vi "HFRR ADV v06.vi"() -> ()   [LabVIEW 2025] (continued)
1.510957261467722, 1.5101897326343034, 1.5103432384009872, 1.5098827211009362, 1.5114177787677732, 1.5108037557010383, 1.5104967441676709, 1.510957261467722, 1.5101897326343034, 1.5111107672344057, 1.5106502499343546, 1.5103432384009872, 1.5108037557010383, 1.5095757095675688, 1.5106502499343546, 1.5103432384009872, 1.5104967441676709, 1.5111107672344057, 1.5104967441676709, 1.5103432384009872, 1.5112642730010895, 1.5108037557010383, 1.5103432384009872, 1.5104967441676709, 1.5106502499343546, 1.5106502499343546, 1.5108037557010383, 1.5111107672344057, 1.5095757095675688, 1.5097292153342525, 1.5111107672344057, 1.5104967441676709, 1.5138738710347124, 1.5138738710347124, 1.5124923191345592, 1.5115712845344569, 1.510957261467722, 1.509422203800885, 1.5108037557010383, 1.5104967441676709, 1.5101897326343034, 1.5104967441676709, 1.5101897326343034, 1.5101897326343034, 1.5103432384009872, 1.5101897326343034, 1.5104967441676709, 1.5101897326343034, 1.5108037557010383, 1.5106502499343546, 1.5098827211009362, 1.5112642730010895, 1.5098827211009362, 1.510957261467722, 1.5104967441676709, 1.5101897326343034, 1.5101897326343034, 1.5103432384009872, 1.5108037557010383, 1.5097292153342525, 1.5111107672344057, 1.5108037557010383, 1.5104967441676709, 1.5112642730010895, 1.5103432384009872, 1.5097292153342525, 1.5104967441676709, 1.5106502499343546, 1.5108037557010383, 1.5100362268676197, 1.5106502499343546, 1.5106502499343546, 1.5103432384009872, 1.5097292153342525, 1.5106502499343546, 1.5100362268676197, 1.5111107672344057, 1.5108037557010383, 1.5100362268676197, 1.5101897326343034, 1.5117247903011406, 1.5117247903011406, 1.510957261467722, 1.5100362268676197, 1.510957261467722, 1.5112642730010895, 1.5103432384009872, 1.5112642730010895, 1.5098827211009362, 1.5112642730010895, 1.510957261467722, 1.5106502499343546, 1.5123388133678755, 1.5123388133678755, 1.5103432384009872, 1.5101897326343034, 1.5101897326343034, 1.5104967441676709, 1.5097292153342525, 1.5111107672344057, 1.5108037557010383, 1.5126458249012429, 1.5117247903011406, 1.5100362268676197, 1.5106502499343546, 1.5098827211009362, 1.5104967441676709, 1.5098827211009362, 1.5106502499343546, 1.5115712845344569, 1.5108037557010383, 1.5112642730010895, 1.5100362268676197, 1.5112642730010895, 1.5104967441676709, 1.5098827211009362, 1.5091151922675177, 1.5112642730010895, 1.5103432384009872, 1.514641399868131, 1.5154089287015495, 1.5117247903011406, 1.5111107672344057, 1.5101897326343034, 1.5098827211009362, 1.5106502499343546, 1.5106502499343546, 1.5106502499343546, 1.5106502499343546, 1.5104967441676709, 1.5112642730010895, 1.5103432384009872, 1.5108037557010383, 1.5106502499343546, 1.5097292153342525, 1.510957261467722, 1.5112642730010895, 1.5103432384009872, 1.510957261467722, 1.5112642730010895, 1.5111107672344057, 1.5106502499343546, 1.5097292153342525, 1.5101897326343034, 1.5097292153342525, 1.5114177787677732, 1.5100362268676197, 1.5103432384009872, 1.5114177787677732, 1.5104967441676709, 1.5112642730010895, 1.5108037557010383, 1.509422203800885, 1.5108037557010383, 1.510957261467722, 1.5108037557010383, 1.5108037557010383, 1.5106502499343546, 1.5108037557010383, 1.510957261467722, 1.5117247903011406, 1.5092686980342014, 1.5098827211009362, 1.5108037557010383, 1.5104967441676709, 1.510957261467722, 1.5111107672344057, 1.5114177787677732, 1.5114177787677732, 1.5114177787677732, 1.5100362268676197, 1.509422203800885, 1.5114177787677732, 1.5106502499343546, 1.5100362268676197, 1.5108037557010383, 1.5103432384009872, 1.5108037557010383, 1.510957261467722, 1.5101897326343034, 1.5103432384009872, 1.5098827211009362, 1.5114177787677732, 1.5108037557010383, 1.5104967441676709, 1.510957261467722, 1.5101897326343034, 1.5111107672344057, 1.5106502499343546, 1.5103432384009872, 1.5108037557010383, 1.5095757095675688, 1.5106502499343546, 1.5103432384009872, 1.5104967441676709, 1.5111107672344057, 1.5104967441676709, 1.5103432384009872, 1.5112642730010895, 1.5108037557010383, 1.5103432384009872, 1.5104967441676709, 1.5106502499343546, 1.5106502499343546, 1.5108037557010383, 1.5111107672344057, 1.5095757095675688, 1.5097292153342525, 1.5111107672344057, 1.5104967441676709, 1.5138738710347124, 1.5138738710347124, 1.5124923191345592, 1.5115712845344569, 1.510957261467722, 1.509422203800885, 1.5108037557010383, 1.5104967441676709, 1.5101897326343034, 1.5104967441676709, 1.5101897326343034, 1.5101897326343034, 1.5103432384009872, 1.5101897326343034, 1.5104967441676709, 1.5101897326343034, 1.5108037557010383, 1.5106502499343546, 1.5098827211009362, 1.5112642730010895, 1.5098827211009362, 1.510957261467722, 1.5104967441676709, 1.5101897326343034, 1.5101897326343034, 1.5103432384009872, 1.5108037557010383, 1.5097292153342525, 1.5111107672344057, 1.5108037557010383, 1.5104967441676709, 1.5112642730010895, 1.5103432384009872, 1.5097292153342525, 1.5104967441676709, 1.5106502499343546, 1.5108037557010383, 1.5100362268676197, 1.5106502499343546, 1.5106502499343546, 1.5103432384009872, 1.5097292153342525, 1.5106502499343546, 1.5100362268676197, 1.5111107672344057, 1.5108037557010383, 1.5100362268676197, 1.5101897326343034, 1.5117247903011406, 1.5117247903011406, 1.510957261467722, 1.5100362268676197, 1.510957261467722, 1.5112642730010895, 1.5103432384009872, 1.5112642730010895, 1.5098827211009362, 1.5112642730010895, 1.510957261467722, 1.5106502499343546, 1.5123388133678755, 1.5123388133678755, 1.5103432384009872, 1.5101897326343034, 1.5101897326343034, 1.5104967441676709, 1.5097292153342525, 1.5111107672344057, 1.5108037557010383, 1.5126458249012429, 1.5117247903011406, 1.5100362268676197, 1.5106502499343546, 1.5098827211009362, 1.5104967441676709, 1.5098827211009362, 1.5106502499343546, 1.5115712845344569, 1.5108037557010383, 1.5112642730010895, 1.5100362268676197, 1.5112642730010895, 1.5104967441676709, 1.5098827211009362, 1.5091151922675177, 1.5112642730010895, 1.5103432384009872, 1.514641399868131, 1.5154089287015495, 1.5117247903011406, 1.5111107672344057, 1.5101897326343034, 1.5098827211009362, 1.5106502499343546, 1.5106502499343546, 1.5106502499343546, 1.5106502499343546, 1.5104967441676709, 1.5112642730010895, 1.5103432384009872, 1.5108037557010383, 1.5106502499343546, 1.5097292153342525, 1.510957261467722, 1.5112642730010895, 1.5103432384009872, 1.510957261467722, 1.5112642730010895, 1.5111107672344057, 1.5106502499343546, 1.5097292153342525, 1.5101897326343034, 1.5097292153342525, 1.5114177787677732, 1.5100362268676197, 1.5103432384009872, 1.5114177787677732, 1.5104967441676709, 1.5112642730010895, 1.5108037557010383, 1.509422203800885, 1.5108037557010383, 1.510957261467722, 1.5108037557010383, 1.5108037557010383, 1.5106502499343546, 1.5108037557010383, 1.510957261467722, 1.5117247903011406, 1.5092686980342014, 1.5098827211009362, 1.5108037557010383, 1.5104967441676709, 1.510957261467722, 1.5111107672344057, 1.5114177787677732, 1.5114177787677732, 1.5114177787677732, 1.5100362268676197, 1.509422203800885, 1.5114177787677732, 1.5106502499343546, 1.5100362268676197, 1.5108037557010383, 1.5103432384009872, 1.5108037557010383, 1.510957261467722, 1.5101897326343034, 1.5103432384009872, 1.5098827211009362, 1.5114177787677732, 1.5108037557010383, 1.5104967441676709, 1.510957261467722, 1.5101897326343034, 1.5111107672344057, 1.5106502499343546, 1.5103432384009872, 1.5108037557010383, 1.5095757095675688, 1.5106502499343546, 1.5103432384009872, 1.5104967441676709, 1.5111107672344057, 1.5104967441676709, 1.5103432384009872, 1.5112642730010895, 1.5108037557010383, 1.5103432384009872, 1.5104967441676709, 1.5106502499343546, 1.5106502499343546, 1.5108037557010383, 1.5111107672344057, 1.5095757095675688, 1.5097292153342525, 1.5111107672344057, 1.5104967441676709, 1.5138738710347124, 1.5138738710347124, 1.5124923191345592, 1.5115712845344569, 1.510957261467722, 1.509422203800885, 1.5108037557010383, 1.5104967441676709, 1.5101897326343034, 1.5104967441676709, 1.5101897326343034, 1.5101897326343034, 1.5103432384009872, 1.5101897326343034, 1.5104967441676709, 1.5101897326343034, 1.5108037557010383, 1.5106502499343546, 1.5098827211009362, 1.5112642730010895, 1.5098827211009362, 1.510957261467722, 1.5104967441676709, 1.5101897326343034, 1.5101897326343034, 1.5103432384009872, 1.5108037557010383, 1.5097292153342525, 1.5111107672344057, 1.5108037557010383, 1.5104967441676709, 1.5112642730010895, 1.5103432384009872, 1.5097292153342525, 1.5104967441676709, 1.5106502499343546, 1.5108037557010383, 1.5100362268676197, 1.5106502499343546, 1.5106502499343546, 1.5103432384009872, 1.5097292153342525, 1.5106502499343546, 1.5100362268676197, 1.5111107672344057, 1.5108037557010383, 1.5100362268676197, 1.5101897326343034, 1.5117247903011406, 1.5117247903011406, 1.510957261467722, 1.5100362268676197, 1.510957261467722, 1.5112642730010895, 1.5103432384009872, 1.5112642730010895, 1.5098827211009362, 1.5112642730010895, 1.510957261467722, 1.5106502499343546, 1.5123388133678755, 1.5123388133678755, 1.5103432384009872, 1.5101897326343034, 1.5101897326343034, 1.5104967441676709, 1.5097292153342525, 1.5111107672344057, 1.5108037557010383, 1.5126458249012429, 1.5117247903011406, 1.5100362268676197, 1.5106502499343546, 1.5098827211009362, 1.5104967441676709, 1.5098827211009362, 1.5106502499343546, 1.5115712845344569, 1.5108037557010383, 1.5112642730010895, 1.5100362268676197, 1.5112642730010895, 1.5104967441676709, 1.5098827211009362, 1.5091151922675177, 1.5112642730010895, 1.5103432384009872, 1.514641399868131, 1.5154089287015495, 1.5117247903011406, 1.5111107672344057, 1.5101897326343034, 1.5098827211009362, 1.5106502499343546, 1.5106502499343546, 1.5106502499343546, 1.5106502499343546, 1.5104967441676709, 1.5112642730010895, 1.5103432384009872, 1.5108037557010383, 1.5106502499343546, 1.5097292153342525, 1.510957261467722, 1.5112642730010895, 1.5103432384009872, 1.510957261467722, 1.5112642730010895, 1.5111107672344057, 1.5106502499343546, 1.5097292153342525, 1.5101897326343034, 1.5097292153342525, 1.5114177787677732, 1.5100362268676197, 1.5103432384009872, 1.5114177787677732, 1.5104967441676709, 1.5112642730010895, 1.5108037557010383, 1.509422203800885, 1.5108037557010383, 1.510957261467722, 1.5108037557010383, 1.5108037557010383, 1.5106502499343546, 1.5108037557010383, 1.510957261467722, 1.5117247903011406, 1.5092686980342014, 1.5098827211009362, 1.5108037557010383, 1.5104967441676709, 1.510957261467722, 1.5111107672344057, 1.5114177787677732, 1.5114177787677732, 1.5114177787677732, 1.5100362268676197, 1.509422203800885, 1.5114177787677732, 1.5106502499343546, 1.5100362268676197, 1.5108037557010383, 1.5103432384009872, 1.5108037557010383, 1.510957261467722, 1.5101897326343034, 1.5103432384009872, 1.5098827211009362, 1.5114177787677732, 1.5108037557010383, 1.5104967441676709, 1.510957261467722, 1.5101897326343034, 1.5111107672344057, 1.5106502499343546, 1.5103432384009872, 1.5108037557010383, 1.5095757095675688, 1.5106502499343546, 1.5103432384009872, 1.5104967441676709, 1.5111107672344057, 1.5104967441676709, 1.5103432384009872, 1.5112642730010895, 1.5108037557010383, 1.5103432384009872, 1.5104967441676709, 1.5106502499343546, 1.5106502499343546, 1.5108037557010383, 1.5111107672344057, 1.5095757095675688, 1.5097292153342525, 1.5111107672344057, 1.5104967441676709, 1.5138738710347124, 1.5138738710347124, 1.5124923191345592, 1.5115712845344569, 1.510957261467722, 1.509422203800885, 1.5108037557010383, 1.5104967441676709, 1.5101897326343034, 1.5104967441676709, 1.5101897326343034, 1.5101897326343034, 1.5103432384009872, 1.5101897326343034, 1.5104967441676709, 1.5101897326343034, 1.5108037557010383, 1.5106502499343546, 1.5098827211009362, 1.5112642730010895, 1.5098827211009362, 1.510957261467722, 1.5104967441676709, 1.5101897326343034, 1.5101897326343034, 1.5103432384009872, 1.5108037557010383, 1.5097292153342525, 1.5111107672344057, 1.5108037557010383, 1.5104967441676709, 1.5112642730010895, 1.5103432384009872, 1.5097292153342525, 1.5104967441676709, 1.5106502499343546, 1.5108037557010383, 1.5100362268676197, 1.5106502499343546, 1.5106502499343546, 1.5103432384009872, 1.5097292153342525, 1.5106502499343546, 1.5100362268676197, 1.5111107672344057, 1.5108037557010383, 1.5100362268676197, 1.5101897326343034, 1.5117247903011406, 1.5117247903011406, 1.510957261467722, 1.5100362268676197, 1.510957261467722, 1.5112642730010895, 1.5103432384009872]
  out "Numeric":i32=178
  out "Flag":dbl format="%.2f"
  in  "Tab Control 3":enum32{"RMS", "LIVE"}(tab)
  out "array w/ subset deleted":dbl[](array[numeric])
  out "REMARKS":string="@WINDUCOM : RECIPROCATORY TEST RIG    DEFINITON FILE       \r  Sample ID :- , Load :-  2.00 N , Remarks :- , Date :- 05/11/2016, 06:04\r"
  out "Time 2":dbl=0.0004
  in  "reinit":bool=TRUE
  in  "Remarks : 2":string
  out "Err Count":i32
  out "PID-out":dbl
  out "Rate":dbl=2500.0 caption="Rate (Hz)" min=100.0 max=10000.0 step=1.0
  out "COUNT":i32
  out "FRICVALZ":dbl
  out "Sensor mean 3":dbl
  out "Sensor mean":dbl(slide) min=0.0 max=5.0 step=0.001 scale=0.0..5.0
  out "Sensor mean 2":dbl
  in  "ao0":errorcluster
  out "String 2":string
  out "clk":dbl min=0.0 max=999999999.0 step=0.25 format="%.2f"
  out "spm":string
  out "stp":dbl=0.25 min=0.25 max=60.0 step=0.25 format="%.2f"
  # "System Control Commands\nS;1 - Starts the full automation cycle (Runs Priming-humidify till 70RH sequence first, then switches to Maintenance).\nS;0 - Stops the system immediately and enters Standby mode (Safe State: All actuators OFF).\nM;1 - Skips the priming sequence and jumps directly to Maintenance mode (PID control).\nR;1 - Resets the logic state machine and clears all errors, returning to Standby.\nService Mode (Manual Control)\nX;1 - Enters Manual Service Mode. This disables all automatic logic, sensor safety checks, and timers.\nX;0 - Exits Manual Service Mode and returns to Standby (Safe State).\nActuator Commands (Only work after sending X;1)\nP;[0-255] - Sets the Pump PWM. Note that this is Active Low (0 = Max Flow, 255 = Pump OFF).\nF;I;[0-255] - Sets the Intake Fan speed (0 = OFF, 255 = Max Speed).\nF;O;[0-255] - Sets the Exhaust Fan speed (0 = OFF, 255 = Max Speed).\nD;1 - Turns the Dehumidifier Relay ON.\nD;0 - Turns the Dehumidifier Relay OFF."
  # "°"
  # "HFRR adv"
  # "HFRR adv"
  # "Camera Initialization in Progress"
  # "Test Setup"
  # "SAMPLE INFO"
  # "Hz"
  # "N"
  # "mm"
  # "°C"
  # "%RH"
  # "min"
  # "left"
  # "%RH"
  # "°C"
  # "Coefficient of Friction"
  # "Frictional Force ( N )"
  # "Electrical Contact Resistance ( % )"
  # "Temperature ( °C )"
  # "Heater"
  # "( mm )"
  # "Hz"
  # "%Rh"
  # "Stroke ( mm )"
  # "%"
  # "N"
  # "deg C"
  # "N"
  # "Automated Scar Detection in Progress"
  # "Zoom Factor"
  # "%"
  # "Tools"
  # "Wear Scar Measurements"
  # "Wear Scar"
  # "Wear Scar"
  # "Wear Scar"
  # "µm"
  # "µm"
  # "µm"
  # "Data points"
  # "Captured if Stroke is +-0.5 of 1mm"
  # "Stroke calibration Procedure: \n1. Insert step 1 in between pushrod and stud and correct the offeset        value  of high pricision laser displacement sensor and the software value.\n2. Insert step 2 (of 0.5mm) and press the capture button to enter\nthe readings in the table shown below\n3. Follow the procedure 3 times and capture the values in  the table.\n4. Press Calculate button to read the error in the gain value."
  # "Calibration assembly image"
  # "ISO : WS1.4"
  # "Reference Fluid Information"
  # "Note:\nMake sure to place all images in the folder \"C:\\WinDucom\\im\" before clicking on \"Import Image.\""
  # "LAB-IQ-NXT\\ WO 2464 \\ v02 \\ DECEMBER 2025"
  # "NOTE:\nPlace all the images in the path \"C:\\WinDucom\\im\" before clicking on Import Image"
  # "Wear Scar Measurements"
  # "Reference Fluid Information"
  # "Graph :"
types:
  T1 = enum32{"Home", "Dashboard", "Imaging", "Report", "Analysis", "About", "Test Setup"}
  T2 = enum32{"HOME", "Test Setup", "Acquire", "Adv Scar", "Adv Scar Report", "Compare Files", "About", "Advance", "Mooha"}
  T3 = enum16{"ASTM D6079", "ISO 12156", "CEC F-096-A-06", "Custom"}
  T4 = enum32{"Dashboard 1", "Dashboard 2", "Dashboard 3"}
  T5 = enum32{"COF", "Friction", "ECR", "Temperature", "Humidity", "Stroke"}
  T6 = enum32{"Coefficient Of Friction", "Air Temperature", "Humidity", "Stroke", "Sample Temperature", "Electrical Contact Resistance", "Frequency", "Air Temp vs Rh"}
  T7 = enum32{"Stroke Data", "Temperature Calibration", "Friction Force Raw Data"}
  T8 = cluster{"Proportional Gain (Kc)":dbl, "Integral Time (Ti, min)":dbl, "Derivative Time (Td, min)":dbl}
  T9 = enum32{"Freqz control", "Low Speed Analog Inputs & Digital IOs", "Temperature Tuning", "Voltage LVDT raw", "High Speed Analog Inputs - Displacement & Friction", "LVDT Calibration", "Sericve", "Friction Force Calibration", "Bytes At Port", "Loadcell Board"}
  T10 = cluster{"proportional gain (Kc)":dbl, "integral time (Ti, min)":dbl, "derivative time (Td, min)":dbl}
  T11 = typedef "imagedata.ctl" = cluster{"image type":i32, "image depth":i32, "image":u8[], "mask":u8[], "colors":u32[], "Rectangle":cluster{"left":i16, "top":i16, "right":i16, "bottom":i16}}
  T12 = enum32{"HOME", "Test Setup", "Acquire", "Compare Files", "Print Report", "About", "Advance", "Mooha"}
  T13 = cluster{"Read Heave and Surge":string, "Bytes at Heave Port":dbl, "Heave and Surge COM Port:":refnum<visa-resource-name>, "Com Port 2":refnum<visa-resource-name>, "Residual Due":string, "Heave COM Status 2":bool, "Heave COM Status":bool, "Port 2":bool, "Sway PPR":dbl, "Surge PPR":dbl, "Heave PPR":dbl, "Sway Pitch":dbl, "Surge Pitch":dbl, "Heave Pitch":dbl, "Sway Pulses/mm":dbl, "Surge Pulses/mm":dbl, "Heave Pulses/mm":dbl, "inner loop":dbl, "Read Heave and Surge 2":string, "String 36":string, "Write S":bool, "WriteCC1":string[], "Heave COM Loop":i32, "LastCom":string, "EXIT":bool, "Error Heave":errorcluster}
  T14 = enum8{"Enabled", "Disabled", "Disabled and Grayed Out"}
  T15 = typedef "POST ANALYSIS ENUM.ctl" = enum16{"OPEN EXE", "INIT", "OPEN FILE", "FIT", "DRAW REC", "DRAW LINE", "PAN", "ZOOM IN", "ZOOM OUT", "SET ZOOM", "CLEAR ROI", "GET MEASUREMENTS", "RESIZE MODE", "STREAM START", "STREAM STOP", "SHOW UI", "MINIMIZE UI", "HIDE UI", "CKISE APP", "CLOSE CONNECTION", "SAVE IMAGE", "SET ROI COLOR", "READ", "TCP CHECK", "CLOSE"}
  T16 = typedef "CAMERA LIVE FEED ENUM.ctl" = enum16{"OPEN EXE", "INIT", "READ", "CAMERA CONNECT", "CAMERA START", "CAMERA STOP", "CAMERA GRAY", "CAMERA RGB", "CAMERA MINIMIZE", "CAMERA CLOSE", "CAMERA MODE LIST", "CAMERA MODE SET", "CAMERA RESTORE", "CAMERA SAVE", "CLOSE"}
  T17 = cluster{"File Name":string, "Test Method":string, "Operator":string, "Fuel Description":string, "Date and time":string}
  T18 = enum32{"HOME", "Test Setup", "Acquire", "Compare Files", "About", "Advance", "Mooha"}
  T19 = enum16{"deny read/write", "deny write-only", "deny none"}
  T20 = typedef "NI_ReportGenerationCore.lvlib/HTML Report Image Alignment.ctl" = enum16{"(default)", "LEFT", "RIGHT", "TOP", "TEXTTOP", "MIDDLE", "ABSMIDDLE", "BASELINE", "BOTTOM", "ABSBOTTOM"}
  T21 = enum16{"open", "replace", "create", "open or create", "replace or create", "replace or create with confirmation"}
  T22 = enum16{"INIT", "READ", "MANUAL WRITE", "WRITE", "CLOSE", "ERROR INIT"}
  T23 = enum16{"open", "open or create", "create or replace", "create", "open (read only)"}
  T24 = cluster{"Mode":enum16{"RTU", "ASCII"}, "Slave Address":u8}
diagram:
  w4 = FALSE ("Humidity Off Command")
  w19 = "" ("USER ID")
  # "[CH1]    - FF\n[CH2]   - TEMPERATURE\n[CH3]    - Humidity\n[CH4]    - AIR TEMP\n[CH5]\\- Visa Uno\n[CH6] \\- Visa Due\n[CH7]  \\- file path\n[CH8]   - Displacement Gain\n[CHA]   - Stroke Gain\n[CHB]   - Stroke PID Gain\n[CHC]   -Language Selection\n[CHD]   -Power +\n[CHE]   -Power_\n[CHF]   -Heater\n[CHG]   -Humidity Wet\n[CHH]   -Humidity Dry\n[CHI]   -Integral Time \n[CHIJ   -Air intercept\n[CHI]   -Temp Intercept"
  n1 = flat-sequence {
    tunnel: [w57] -> w9
    tunnel: w9 -> [w71]
    tunnel: [w70] -> w8
    tunnel: ["ao0"] -> w11
    tunnel: w8 -> [_]
    tunnel: w11 -> [w136]
    tunnel: [w136] -> w10
    tunnel: w10 -> [w189]
    tunnel: [w187] -> w23
    tunnel: [w189] -> w22
    tunnel: w23 -> [w240]
    tunnel: w22 -> [w196]
    tunnel: [w240] -> w7
    tunnel: [w202] -> w6
    tunnel: [w190] -> w5
    tunnel: [w247] -> _
    tunnel: [w246] -> _
    tunnel: [w248] -> w51
    tunnel: w7 -> [w248]
    tunnel: w6 -> [w246]
    tunnel: w5 -> [w247]
    frame #0 {
      n2 = call "CLOSE CONNECTION.vi"("error in (no error)"="error in (no error) 2") -> ("error out"=w55:errorcluster)  [unwired: 10 in]
      n3 = call <vilib>:"Clear Errors.vi"("error in (no error)"=w55) -> ("error out"=w54:errorcluster)  [unwired: 5 in, 1 out]
      n4 = disable-structure shown="Enabled" {
        disable-tunnel: w54 -> [w61 _]
        disable-tunnel: [w60 _] -> w57
        frame Enabled {
          n5 = call <userlib>:"Fit VI window to Largest Dec.vi"("error in (no error)"=w61, "border spacing (2 px)"=1) -> ("error out"=w64:errorcluster, "dup VI Ref"=w68:refnum<vi>)  [unwired: 4 in]
          n6 = invoke on="Invoke Node" class="VI" method="FP.Run-Time Position.Maximized"(reference=w68, error in=w64) -> (error out=w65:errorcluster)  [unwired: 2 in, 3 out]
          n7 = call <vilib>:"Clear Errors.vi"("error in (no error)"=w65) -> ("error out"=w67:errorcluster)  [unwired: 5 in, 1 out]
          n8 = control-ref of="This VI"() -> (w59:refnum<vi>)
          n9 = invoke on="Invoke Node" class="VI" method="Default Vals.Reinit All"(reference=w59, error in=w67) -> (reference out=w63:refnum<vi>, error out=w62:errorcluster)  [unwired: 1 in, 1 out]
          n10 = Close Reference(reference=w63, error in (no error)=w62) -> (error out=w60:errorcluster)
        }
        frame Disabled {
        }
      }
      n11 = local write "sign in temp"(FALSE ("sign in temp")) -> ()
      n12 = property on="Sign In" class="Bool (strict)"("DisabledEnum"=T14."Disabled" ("Disabled")) -> ()  [unwired: 2 in, 2 out]
      n13 = property on="Auto Scar Check" class="Clust (strict)"("Visible"=TRUE) -> ()  [unwired: 2 in, 2 out]
    }
    frame #1 {
      n14 = call "dialog box.vi"("Status"="Before starting the test, verify that the microscope cable is connected.", "error in"=w71) -> ("error out"=w70:errorcluster)  [unwired: 8 in]
    }
    frame #2 {
      w78 = FALSE ("Upld AR 2")
      # "kkkkk"
      # "C:\\Windows\\wndcm_pw_stdED hfrr.txt"
      # "C:\\LAB-IQ NXT"
      # "C:\\LAB-IQ NXT\\wndcm_pw_stdED hfrr.txt"
      # "password file"
      n15 = Current VI's Path() -> (path=w91:path)
      n16 = Strip Path(path=w91) -> (stripped path=w84:path)  [unwired: 1 out]
      n17 = Path To String(path=w84) -> (string=w86:string)
      n18 = local write "conststatus"(0.0 ("rpm value : 2")) -> ()
      n19 = local write "Upld AR 2"(TRUE ("Upld AR 2")) -> ()
      n20 = local write "Lan flag"(0.0 ("Lan flag")) -> ()
      n21 = local write "COUNT"(0 ("COUNT")) -> ()
      n22 = local write "FLAG 2"(0.0 ("FLAG 2")) -> ()
      n23 = local write "Com flag"(u32 0 ("Com flag")) -> ()
      n24 = local write "Re-Initialise"(TRUE ("Re-Initialise")) -> ()
      n25 = local write "refresh flag"(FALSE ("refresh flag")) -> ()
      n26 = local write "Json St Flg"(w78) -> ()
      n27 = Search/Split String(string=w86, search string/char (-)=".exe") -> (match + rest of string=w88:string)  [unwired: 1 in, 2 out]
      n28 = Match True/False String(2:".vi" ("false string"), 3:".exe" ("true string"), 4:w88) -> (0:w85:bool)  [unwired: 1 out]
      n29 = local write "Json End Flg"(w78) -> ()
      n30 = case shown="True" w85 {
        tunnel: w84 -> [w107 w109]
        tunnel: [w107 w108] -> w82
        frame False {
        }
        frame True {
          n31 = Strip Path(path=w109) -> (stripped path=w108:path)  [unwired: 1 out]
        }
      }
      n32 = Path To String(path=w82) -> (string=→"Gain path":string)
      n33 = local write "Main Tab Display"(T4."Dashboard 1" ("Main Tab Display")) -> ()
      n34 = local write "main tab sub"(enum32{"Page 1", "Page 2"}."Page 1" ("main tab sub")) -> ()
      n35 = local write "Main Tab"(T2."HOME" ("Main Tab")) -> ()
      n36 = local write "EVENT LOG"("") -> ()
      n37 = List Folder(path=path "C:/LAB-IQ" ("directory path"), pattern="*.txt") -> (filenames=w97:string[])  [unwired: 2 in, 3 out]
      n38 = Search 1D Array(1D array=w97, element="wndcm_pw_stdED hfrr.txt") -> (index of element=w100:i32)  [unwired: 1 in]
      n39 = Equal?(x=w100, y=-1) -> (x = y?=w95:bool)
      n40 = case shown="True" w95 {
        frame False {
        }
        frame True {
          n41 = String To Byte Array(string="123\n") -> (unsigned byte array=w114:u8[])
          n42 = Array Size(array=w114) -> (size(s)=w113:i32)
          n43 = for {
            N: w113 -> [_]
            tunnel: w114 -> [w127]
            tunnel: [w124] -> w116 mode=indexing
            tunnel: w113 -> [w119]
            i -> [w117]
            n44 = Decrement(x=w119) -> (x-1=w120:i32)
            n45 = Equal?(x=w117, y=w120) -> (x = y?=w121:bool)
            n46 = Index Array(array=w127, index=w117) -> (element=w126:u8)
            n47 = Number To Decimal String(number=w126) -> (decimal integer string=w125:string)  [unwired: 1 in]
            n48 = Select(t="", s=w121, f="\r") -> (s? t:f=w118:string)
            n49 = Concatenate Strings(w125, w118) -> (w124:string)
          }
          n50 = local read "file path"() -> (w110:path)
          n51 = Concatenate Strings(w116) -> (w112:string)
          n52 = call <vilib>:"Write Characters To File.vi"("append to file? (new file:F)"=FALSE, "character string"=w112, "file path (dialog if empty)"=w110) -> ()  [unwired: 2 in, 1 out]
        }
      }
      n53 = local write "clk"(0.0 ("clk")) -> ()
      n54 = local write "Flag"(0.0 ("Flag")) -> ()
      "file path" <- path "C:/LAB-IQ/wndcm_pw_stdED hfrr.txt" ("file path")
      "FF buffer" <- dbl[] [] ("FF buffer")
    }
    frame #3 {
      # "C:\\WinDucom\\calibrate WO 2391.dcf"
      n55 = String To Path(string="C:\\LAB-IQ\\calibrate WO 2464.dcf") -> (path=w135:path)
      n56 = Open/Create/Replace File "Open File"(file path (use dialog)=w135) -> (refnum out=w134:refnum<file>)  [unwired: 5 in, 2 out]
      n57 = for {
        N: 24 -> [_]
        tunnel: w134 -> [w155]
        i -> [w149]
        (unwired) TRUE ("line mode (F)")
        n58 = Read from Text File "Read File"(file (use dialog)=w155) -> (text=w154:string)  [unwired: 3 in, 3 out]
        n59 = Match Pattern(string=w154, regular expression="]") -> (after substring=w152:string)  [unwired: 1 in, 3 out]
        n60 = String Subset(string=w154, offset (0)=5, length (rest)=10 ("length (rest)")) -> (substring=w147:string)
        n61 = Fract/Exp String To Number(string=w147) -> (number=w148:dbl)  [unwired: 3 in, 1 out]
        n62 = Match Pattern(string=w152, regular expression="-") -> (before substring=w150:string)  [unwired: 1 in, 3 out]
        n63 = case shown="6" w149 {
          tunnel: w148 -> [w158 w159 w160 w161 _ _ _ w166 w167 w168 w171 w172 w173 w174 w175 w176 w177 w180 w181 _ _ w184 _ _ _]
          tunnel: w150 -> [_ _ _ _ w162 w163 w164 _ _ _ _ _ _ _ _ _ _ _ _ w182 w183 _ w185 w186 _]
          frame 0 {
            n64 = local write "FRIC. FORCE :"(w158) -> ()
          }
          frame 1 {
            n65 = local write "TEMPERATURE :"(w159) -> ()
          }
          frame 2 {
            n66 = local write "HUMIDITY:"(w160) -> ()
          }
          frame 3 {
            n67 = local write "AIR TEMPERATURE :"(w161) -> ()
          }
          frame 4 {
            n68 = local write "Com Port 1"(w162) -> ()
          }
          frame 5 {
            n69 = local write "Com Port 2"(w163) -> ()
            n70 = local write "visa due"(w163) -> ()
          }
          frame 6 {
            n71 = String To Path(string=w164) -> (path=w165:path)
            n72 = local write "File Path"(w165) -> ()
          }
          frame 7 {
            n73 = local write "DISPLACEMENT :"(w166) -> ()
          }
          frame 8 {
            n74 = local write "STROKE GAIN :"(w167) -> ()
          }
          frame 9 {
            n75 = local read "Stroke PID Gains"() -> (w170:T8)
            n76 = Bundle By Name(cluster=w170, "Proportional Gain (Kc)"=w168) -> (w169:T8)
            n77 = local write "Stroke PID Gains"(w169) -> ()
          }
          frame 10 {
            n78 = local write "Language Selection"(w171) -> ()
          }
          frame 11 {
            n79 = local write "CH-POWER +"(w172) -> ()
          }
          frame 12 {
            n80 = local write "CH-POWER -"(w173) -> ()
          }
          frame 13 {
            n81 = local write "CH-HEATER"(w174) -> ()
          }
          frame 14 {
            n82 = local write "CH-HUMIDITY WET"(w175) -> ()
          }
          frame 15 {
            n83 = local write "CH-HUMIDITY DRY"(w176) -> ()
          }
          frame 16 {
            n84 = local read "Stroke PID Gains"() -> (w179:T8)
            n85 = Bundle By Name(cluster=w179, "Integral Time (Ti, min)"=w177) -> (w178:T8)
            n86 = local write "Stroke PID Gains"(w178) -> ()
          }
          frame 17 {
            n87 = local write "AIR TEMP INTERCEPT:"(w180) -> ()
          }
          frame 18 {
            n88 = local write "TEMP INTERCEPT:"(w181) -> ()
          }
          frame 19 {
            n89 = local write "S.NO"(w182) -> ()
          }
          frame 20 {
            n90 = local write "Com Port 3"(w183) -> ()
          }
          frame 21 {
            n91 = local write "LvdtOff"(w184) -> ()
          }
          frame 22 {
            n92 = local write "Humidity :"(w185) -> ()
          }
          frame 23 {
            n93 = local write "Camera Port :"(w186) -> ()
          }
          frame 24, Default {
          }
        }
      }
      n94 = String To Path(string="C:\\LAB-IQ\\Image Calibrate v01.dcf") -> (path=w131:path)
      n95 = Open/Create/Replace File ("Open File")(file path (use dialog)=w131) -> (refnum out=w130:refnum<file>)  [unwired: 5 in, 2 out]
      n96 = for {
        N: 4 -> [_]
        tunnel: w130 -> [w142]
        i -> [w138]
        n97 = Read from Text File ("Read File")(file (use dialog)=w142) -> (text=w143:string)  [unwired: 3 in, 3 out]
        n98 = String Subset(string=w143, offset (0)=6, length (rest)=10 ("length (rest)")) -> (substring=w139:string)
        n99 = Fract/Exp String To Number(string=w139) -> (number=w137:dbl)  [unwired: 3 in, 1 out]
        n100 = case shown="3" w138 {
          tunnel: w137 -> [w144 w145 _ w146 _]
          frame 0 {
            n101 = local write "5x Gain"(w144) -> ()
          }
          frame 1 {
            n102 = local write "10x Gain"(w145) -> ()
          }
          frame 2 {
          }
          frame 3 {
            n103 = local write "100x gain"(w146) -> ()
          }
          frame 4, Default {
          }
        }
      }
    }
    frame #4 {
      n104 = Wait (ms)(milliseconds to wait=u32 1000) -> (millisecond timer value=w187:u32)
    }
    frame #5 {
      w205 = u32 2000 ("milliseconds to wait")
      w232 = u32 3000 ("milliseconds to wait")
      n105 = local read "Re-Initialise"() -> (w239:bool)
      n106 = case shown="True" w239 {
        frame False {
        }
        frame True {
          n107 = local write "Re-Initialise"(FALSE ("Re-Initialise")) -> ()
        }
      }
      n108 = call "CAMERA LIVE FEED FGV.vi"("Enum - Menu"=CAMERA_LIVE_FEED_ENUM."OPEN EXE", "error in (no error)"=w196) -> ("error out"=w238:errorcluster)  [unwired: 8 in, 1 out]
      n109 = call "Stall Data Flow.vim"("value in"=w238, "milliseconds to wait"=w232) -> ("value out"=w236:errorcluster)  [unwired: 1 out]
      n110 = call "CAMERA LIVE FEED FGV.vi"("Enum - Menu"=CAMERA_LIVE_FEED_ENUM."INIT", "error in (no error)"=w236) -> ("error out"=w234:errorcluster)  [unwired: 8 in, 1 out]
      n111 = call "IMAGE ANALYSIS.vi"("Enum"=POST_ANALYSIS_ENUM."OPEN EXE", "error in"=w196) -> ("error out"=w193:errorcluster)  [unwired: 8 in, 1 out]
      n112 = case shown="Error .." w234 {
        selector: w234 -> [w241 _]
        tunnel: [w241 _] -> w233
        frame No Error {
        }
        frame Error {
          n113 = One Button Dialog(message="Camera initialization error.\nPlease Restart the software") -> ()  [unwired: 1 in, 1 out]
        }
      }
      n114 = call "Stall Data Flow.vim"("value in"=w193, "milliseconds to wait"=u32 10000) -> ("value out"=w192:errorcluster)  [unwired: 1 out]
      n115 = property on="Camera Port :" class="CmbBox"() -> ("Strings[]"=w230:string[], "Value"=w231:string)  [unwired: 2 in, 2 out]
      n116 = call "IMAGE ANALYSIS.vi"("Enum"=POST_ANALYSIS_ENUM."INIT", "error in"=w192) -> ("error out"=w190:errorcluster)  [unwired: 8 in, 1 out]
      n117 = Search 1D Array(1D array=w230, element=w231) -> (index of element=w229:i32)  [unwired: 1 in]
      n118 = Type Cast(type=30, x=w229) -> (*(type *) &x=w227:i32)
      n119 = call "Stall Data Flow.vim"("value in"=w233, "milliseconds to wait"=w232) -> ("value out"=w209:errorcluster)  [unwired: 1 out]
      n120 = Add(x=w227, y=48) -> (x+y=w208:i32)
      n121 = call "CAMERA LIVE FEED FGV.vi"("Enum - Menu"=CAMERA_LIVE_FEED_ENUM."CAMERA CONNECT", "error in (no error)"=w209, "CAMERA PORT"=w208) -> ("error out"=w218:errorcluster)  [unwired: 7 in, 1 out]
      n122 = call "Stall Data Flow.vim"("value in"=w218, "milliseconds to wait"=u32 6500) -> ("value out"=w219:errorcluster)  [unwired: 1 out]
      n123 = call "CAMERA LIVE FEED FGV.vi"("Enum - Menu"=CAMERA_LIVE_FEED_ENUM."CAMERA MODE LIST", "error in (no error)"=w219) -> ("error out"=w221:errorcluster)  [unwired: 8 in, 1 out]
      n124 = call "Stall Data Flow.vim"("value in"=w221, "milliseconds to wait"=w205) -> ("value out"=w220:errorcluster)  [unwired: 1 out]
      n125 = Type Cast(type=30, x=0) -> (*(type *) &x=w201:i32)
      n126 = Add(x=w201, y=48) -> (x+y=w199:i32)
      n127 = call "CAMERA LIVE FEED FGV.vi"("Enum - Menu"=CAMERA_LIVE_FEED_ENUM."READ", "error in (no error)"=w220) -> ("error out"=w207:errorcluster, "data out"=→"data out":string)  [unwired: 8 in]
      n128 = call "Stall Data Flow.vim"("value in"=w207, "milliseconds to wait"=w205) -> ("value out"=w206:errorcluster)  [unwired: 1 out]
      n129 = call "CAMERA LIVE FEED FGV.vi"("Enum - Menu"=CAMERA_LIVE_FEED_ENUM."CAMERA MODE SET", "error in (no error)"=w206, "CAMERA MODE"=w199) -> ("error out"=w203:errorcluster)  [unwired: 7 in, 1 out]
      n130 = call "Stall Data Flow.vim"("value in"=w203, "milliseconds to wait"=u32 2000) -> ("value out"=w223:errorcluster)  [unwired: 1 out]
      n131 = call "CAMERA LIVE FEED FGV.vi"("Enum - Menu"=CAMERA_LIVE_FEED_ENUM."CAMERA START", "error in (no error)"=w223) -> ("error out"=w224:errorcluster)  [unwired: 8 in, 1 out]
      n132 = call "Stall Data Flow.vim"("value in"=w224, "milliseconds to wait"=u32 1000) -> ("value out"=w225:errorcluster)  [unwired: 1 out]
      n133 = call "CAMERA LIVE FEED FGV.vi"("Enum - Menu"=CAMERA_LIVE_FEED_ENUM."CAMERA MINIMIZE", "error in (no error)"=w225) -> ("error out"=w202:errorcluster)  [unwired: 8 in, 1 out]
    }
    frame #6 {
      n134 = case shown="No Error" w246 {
        frame No Error {
          n135 = property on="Auto Scar Check" class="Clust (strict)"("Visible"=FALSE) -> ()  [unwired: 2 in, 2 out]
        }
        frame Error {
        }
      }
      n136 = local write "sign in temp"(TRUE ("sign in temp")) -> ()
      n137 = property on="Sign In" class="Bool (strict)"("DisabledEnum"=T14."Enabled" ("Disabled")) -> ()  [unwired: 2 in, 2 out]
    }
  }
  n138 = local write "Temperature Off Command"(w4) -> ()
  n139 = local write "Main Dashboard Buttons"(T1."Home" ("Main Dashboard Buttons")) -> ()
  n140 = local write "Humidity Off Command"(w4) -> ()
  n141 = local write "LIVE FEED MIN TEMP"(w4) -> ()
  n142 = local write "CAMERA ROI MIN TEMP"(w4) -> ()
  n143 = local write "main tab sub"(enum32{"Page 1", "Page 2"}."Page 1" ("main tab sub")) -> ()
  n144 = local write "USERNAME"(w19) -> ()
  n145 = property on="Quit" class="Bool (strict)"("Value"=FALSE ("Quit")) -> (error out=w21:errorcluster)  [unwired: 2 in, 1 out]
  n146 = local write "Main Tab"(T2."HOME" ("Main Tab")) -> ()
  n147 = local write "USER ID"(w19) -> ()
  n148 = while {
    stop <- w274 stop-if-true
    w257 = errorcluster {"status"=FALSE, "code"=0, "source"=""} ("error in (no error) 3")
    # "this loop is for manual report generation"
    n149 = local read "Confirm Measrurement"() -> (w256:bool)
    n150 = case shown="True" w256 {
      selector: w256 -> [_ w348]
      tunnel: errorcluster {"status"=FALSE, "code"=0, "source"=""} ("error in (no error) 3") -> [_ w349]
      tunnel: [_ w347] -> _
      frame False {
      }
      frame True {
        n151 = stacked-sequence {
          tunnel: w349 -> [_ w380 _]
          tunnel: w348 -> [_ _ w457]
          tunnel: [_ w368 _] -> w347
          frame #0 {
            n152 = String To Path(string="C:\\LAB-IQ\\Image Calibrate v01.dcf") -> (path=w352:path)
            n153 = Open/Create/Replace File ("Open File")(file path (use dialog)=w352) -> (refnum out=w353:refnum<file>)  [unwired: 5 in, 2 out]
            n154 = for {
              N: 4 -> [_]
              tunnel: w353 -> [w359]
              i -> [w355]
              n155 = Read from Text File ("Read File")(file (use dialog)=w359) -> (text=w360:string)  [unwired: 3 in, 3 out]
              n156 = String Subset(string=w360, offset (0)=6, length (rest)=10 ("length (rest)")) -> (substring=w356:string)
              n157 = Fract/Exp String To Number(string=w356) -> (number=w354:dbl)  [unwired: 3 in, 1 out]
              n158 = case shown="3" w355 {
                tunnel: w354 -> [w361 w362 _ w363 _]
                frame 0 {
                  n159 = local write "5x Gain"(w361) -> ()
                }
                frame 1 {
                  n160 = local write "10x Gain"(w362) -> ()
                }
                frame 2 {
                }
                frame 3 {
                  n161 = local write "100x gain"(w363) -> ()
                }
                frame 4, Default {
                }
              }
            }
          }
          frame #1 {
            n162 = local read "Magnification :"() -> (w373:string)
            n163 = case shown="\"10x\"" w373 {
              tunnel: [w407 w408] -> w371
              frame "5x", Default {
                n164 = local read "5x Gain"() -> (w407:dbl)
              }
              frame "10x" {
                # "5x"
                n165 = local read "10x Gain"() -> (w408:dbl)
              }
            }
            n166 = call "IMAGE ANALYSIS.vi"("Enum"=POST_ANALYSIS_ENUM."GET MEASUREMENTS", "error in"=w380) -> ("error out"=w387:errorcluster)  [unwired: 8 in, 1 out]
            n167 = call "Stall Data Flow.vim"("value in"=w387, "milliseconds to wait"=u32 1000) -> ("value out"=w386:errorcluster)  [unwired: 1 out]
            n168 = local read "Test File List :"() -> (w384:string)
            n169 = call "IMAGE ANALYSIS.vi"("Enum"=POST_ANALYSIS_ENUM."READ", "error in"=w386) -> ("error out"=w383:errorcluster, "data out"=w374:string)  [unwired: 8 in]
            n170 = Match Pattern(string=w374, regular expression="\"type\": ") -> (after substring=w378:string)  [unwired: 1 in, 3 out]
            n171 = call "IMAGE PATH CREATION PY.vi"("error in (no error)"=w383, "File Name :"=w384) -> ("error out"=w382:errorcluster, "File Path"=w370:path, "File Path String:"=w365:string)  [unwired: 7 in]
            n172 = Match Pattern(string=w378, regular expression=",") -> (before substring=w364:string)  [unwired: 1 in, 3 out]
            n173 = local read "Calibration Tab"() -> (w367:enum32{"Measrument", "Calibrate"})
            n174 = call "Stall Data Flow.vim"("value in"=w382, "milliseconds to wait"=u32 250) -> ("value out"=w366:errorcluster)  [unwired: 1 out]
            n175 = Equal?(x=w364, y="\"rectangle\"") -> (x = y?=w375:bool)
            n176 = case shown="True" w375 {
              tunnel: w374 -> [w413 w454]
              tunnel: w371 -> [_ w445]
              tunnel: cluster{"major":dbl, "minor":dbl, "average":dbl} {"major"=0.0, "minor"=0.0, "average"=0.0} -> [w411 w441]
              tunnel: [w410 w438] -> w369
              tunnel: w364 -> [w412 _]
              tunnel: w371 -> [w409 _]
              frame False {
                n177 = Equal?(x=w412, y="\"line\"") -> (x = y?=w414:bool)
                n178 = case shown="True" w414 {
                  tunnel: w413 -> [_ w424]
                  tunnel: w411 -> [w416 w423]
                  tunnel: [w416 w421] -> w410
                  tunnel: w409 -> [_ w420]
                  frame False {
                  }
                  frame True {
                    w419 = 0.0 ("Major Axis")
                    n179 = Match Pattern(string=w424, regular expression="\"length_px\":") -> (after substring=w422:string)  [unwired: 1 in, 3 out]
                    n180 = Fract/Exp String To Number(string=w422, default (0 dbl)=0.0 ("default (0 DBL)")) -> (number=w417:dbl)  [unwired: 2 in, 1 out]
                    "Pixel Value" <- w417
                    n181 = Multiply(x=w417, y=w420) -> (x*y=w431:dbl)
                    n182 = Multiply(x=w431, y=1000.0) -> (x*y=w418:dbl)
                    n183 = local write "Measurment (mm)"(w418) -> ()
                    n184 = Bundle By Name(cluster=w423, "average"=w418) -> (w421:cluster{"major":dbl, "minor":dbl, "average":dbl})
                    n185 = local write "Average"(w418) -> ()
                    n186 = property on="Major Axis" class="DigNum (strict)"("Caption.Text"="") -> ()  [unwired: 2 in, 2 out]
                    n187 = property on="Minor Axis" class="DigNum (strict)"("Caption.Text"="") -> ()  [unwired: 2 in, 2 out]
                    n188 = property on="Average" class="DigNum (strict)"("Caption.Text"="Line") -> ()  [unwired: 2 in, 2 out]
                    n189 = local write "Minor Axis"(w419) -> ()
                    n190 = local write "Major Axis"(w419) -> ()
                  }
                }
              }
              frame True {
                w442 = 1000.0 ("y")
                w448 = 0.0 ("default (0 DBL)")
                n191 = Match Pattern(string=w454, regular expression=" \"width_px\":") -> (after substring=w452:string)  [unwired: 1 in, 3 out]
                n192 = Match Pattern(string=w452, regular expression="\"height_px\":") -> (before substring=w450:string, after substring=w449:string)  [unwired: 1 in, 2 out]
                n193 = Fract/Exp String To Number(string=w450, default (0 dbl)=w448) -> (number=w447:dbl)  [unwired: 2 in, 1 out]
                n194 = Fract/Exp String To Number(string=w449, default (0 dbl)=w448) -> (number=w446:dbl)  [unwired: 2 in, 1 out]
                n195 = Multiply(x=w447, y=w445) -> (x*y=w444:dbl)
                n196 = Multiply(x=w446, y=w445) -> (x*y=w443:dbl)
                n197 = Multiply(x=w444, y=w442) -> (x*y=w434:dbl)
                n198 = Multiply(x=w443, y=w442) -> (x*y=w433:dbl)
                n199 = Add(x=w434, y=w433) -> (x+y=w440:dbl)
                n200 = property on="Major Axis" class="DigNum (strict)"("Caption.Text"="Major Axis") -> ()  [unwired: 2 in, 2 out]
                n201 = property on="Minor Axis" class="DigNum (strict)"("Caption.Text"="Minor Axis") -> ()  [unwired: 2 in, 2 out]
                n202 = property on="Average" class="DigNum (strict)"("Caption.Text"="Average") -> ()  [unwired: 2 in, 2 out]
                n203 = Divide(x=w440, y=2.0) -> (x/y=w432:dbl)
                n204 = Bundle By Name(cluster=w441, "major"=w434, "minor"=w433, "average"=w432) -> (w438:cluster{"major":dbl, "minor":dbl, "average":dbl})
                n205 = local write "Minor Axis"(w433) -> ()
                n206 = local write "Major Axis"(w434) -> ()
                n207 = local write "Average"(w432) -> ()
              }
            }
            n208 = case shown="\"Measrument\", Default" w367 {
              tunnel: w370 -> [w401 _]
              tunnel: w369 -> [w399 _]
              tunnel: [w391 w406] -> w368
              tunnel: w366 -> [w397 w406]
              tunnel: w365 -> [w396 _]
              frame "Measrument", Default {
                n209 = call "IMAGE ANALYSIS.vi"("Enum"=POST_ANALYSIS_ENUM."SAVE IMAGE", "error in"=w397, "IMAGE FILE PATH"=w396) -> ("error out"=w395:errorcluster)  [unwired: 7 in, 1 out]
                n210 = local read "Test File List :"() -> (w403:string)
                n211 = call "IMAGE ANALYSIS.vi"("Enum"=POST_ANALYSIS_ENUM."MINIMIZE UI", "error in"=w395) -> ("error out"=w393:errorcluster)  [unwired: 8 in, 1 out]
                n212 = Bundle By Name(cluster=T17 {"File Name"="", "Test Method"="", "Operator"="", "Fuel Description"="", "Date and time"=""} ("Main Ref"), "File Name"=w403) -> (w404:T17)
                n213 = call "duf file read.vi"("error in (no error)"=w393, "Main Ref"=w404) -> ("error out"=w402:errorcluster, "Main Ref 2"=w400:T17)  [unwired: 8 in]
                n214 = call "DETECTION REPORT for manual.vi"("error in (no error)"=w402, "return value 3"=w399, "Image File Path"=w401, "Main Ref"=w400) -> ("error out"=w398:errorcluster)  [unwired: 7 in]
                n215 = call "IMAGE ANALYSIS.vi"("Enum"=POST_ANALYSIS_ENUM."SHOW UI", "error in"=w398) -> ("error out"=w391:errorcluster)  [unwired: 8 in, 1 out]
              }
              frame "Calibrate" {
              }
            }
          }
          frame #2 {
            n216 = Not(x=w457) -> (.not. x?=w456:bool)
            n217 = local write "Confirm Measrurement"(w456) -> ()
            n218 = local read "Calibration Tab"() -> (w455:enum32{"Measrument", "Calibrate"})
            n219 = case shown="\"Measrument\", Default" w455 {
              frame "Measrument", Default {
                n220 = local write "Main Tab"(T2."HOME" ("Main Tab")) -> ()
              }
              frame "Calibrate" {
              }
            }
          }
        }
      }
    }
    n221 = local read "Save Change"() -> (w253:bool)
    n222 = local read "Calibrate"() -> (w254:bool)
    n223 = case shown="True" w254 {
      selector: w254 -> [_ w345]
      frame False {
      }
      frame True {
        n224 = Not(x=w345) -> (.not. x?=w344:bool)
        n225 = local write "Calibrate"(w344) -> ()
        n226 = local write "Calibration Tab"(enum32{"Measrument", "Calibrate"}."Calibrate" ("Calibration Tab")) -> ()
      }
    }
    n227 = case shown="True" w253 {
      selector: w253 -> [_ w289]
      frame False {
      }
      frame True {
        n228 = stacked-sequence {
          tunnel: w289 -> [_ _ _ _ w343]
          frame #0 {
            n229 = call "IMAGE ANALYSIS.vi"("Enum"=POST_ANALYSIS_ENUM."HIDE UI") -> ()  [unwired: 9 in, 2 out]
          }
          frame #1 {
            n230 = local read "100x gain"() -> (w291:dbl)
            n231 = local read "10x Gain"() -> (w292:dbl)
            n232 = local read "5x Gain"() -> (w293:dbl)
            n233 = Number To Fractional String(number=w292, width (-)=i16 4, precision (6)=i16 7) -> (F-format string=w314:string)  [unwired: 1 in]
            n234 = Number To Fractional String(number=0.0, width (-)=i16 4, precision (6)=i16 7) -> (F-format string=w309:string)  [unwired: 1 in]
            n235 = Number To Fractional String(number=w291, width (-)=i16 4, precision (6)=i16 7) -> (F-format string=w297:string)  [unwired: 1 in]
            n236 = Number To Fractional String(number=w293, width (-)=i16 10 ("precision (6)"), precision (6)=i16 7) -> (F-format string=w323:string)  [unwired: 1 in]
            n237 = Concatenate Strings("[CH1]" ("string"), w323, " - 5x Gain" ("string"), "\r") -> (w313:string)
            n238 = Concatenate Strings("[CH2]" ("string"), w314, " - 10x Gain" ("string"), "\r") -> (w312:string)
